vi "timings to timings HR.vi"(1 "timing (ms)":T1) -> (0 "String":string)   [LabVIEW 2010, in "slot.xctl"]
uses:
  sequence slot/slot.xctl
  sequence slot/timing.ctl
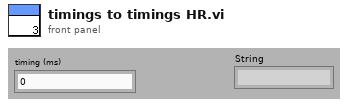
[diagram p1: front panel]
types:
  T1 = typedef "timing.ctl" = sgl
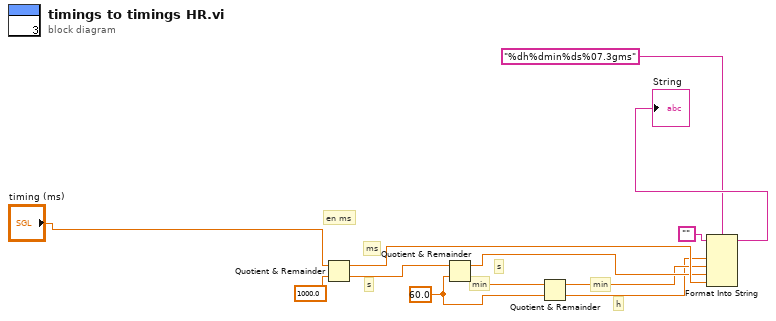
[diagram p0: block diagram]
diagram:
  w4 = 60.0 ("y")
  # "min"
  # "s"
  # "h"
  # "min"
  # "s"
  # "en ms"
  # "ms"
  n1 = Quotient & Remainder(x="timing (ms)", y=1000.0) -> (x-y*floor(x/y)=w12:dbl, floor(x/y)=w7:dbl)
  n2 = Quotient & Remainder(x=w7, y=w4) -> (x-y*floor(x/y)=w11:dbl, floor(x/y)=w8:dbl)
  n3 = Quotient & Remainder(x=w8, y=w4) -> (x-y*floor(x/y)=w10:dbl, floor(x/y)=w9:dbl)
  n4 = Format Into String(format string="%dh%dmin%ds%07.3gms" ("chaîne de format"), initial string="", w9, w10, w11, w12) -> (resulting string=→"String":string)  [unwired: 1 in, 1 out]
